vi "Show State State.vi"(8 "error in (no error)":errorcluster, 9 "State Name":string, 10 "Category (Optional)":string, 11 "JKI SM in":refnum<class "JKI SM.lvclass">) -> (0 "error out":errorcluster, 3 "JKI SM out":refnum<class "JKI SM.lvclass">)   [LabVIEW 2013, in "JKI State Machine API.lvlib" / "JKI SM.lvclass"]
uses:
  JKI SM.lvclass
  JKI SM.lvclass/JKI SM.ctl
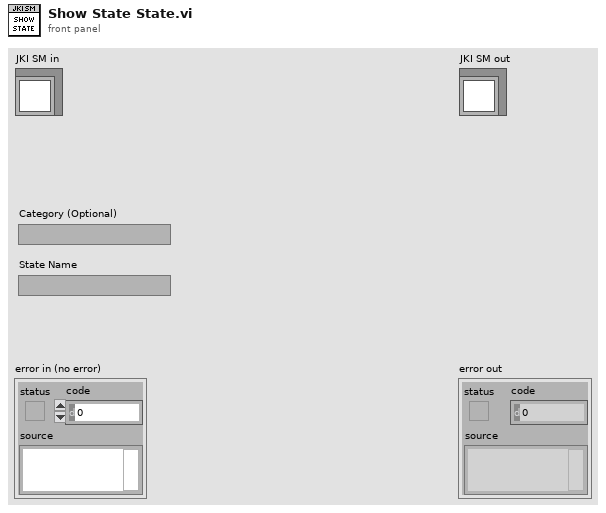
[diagram p1: front panel]
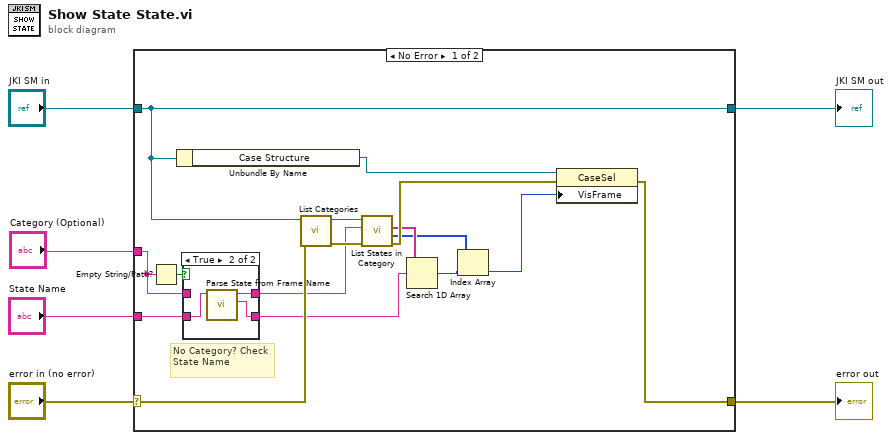
[diagram p0: block diagram]
diagram:
  n1 = case shown="No Error" "error in (no error)" {
    selector: "error in (no error)" -> [w15 w29]
    tunnel: [w22 w29] -> w5
    tunnel: [w16 w28] -> w3
    tunnel: "JKI SM in" -> [w16 w28]
    tunnel: "State Name" -> [w17 _]
    tunnel: "Category (Optional)" -> [w18 _]
    frame No Error {
      # "No Category? Check State Name"
      n2 = Empty String/Path?(string/path=w18) -> (empty?=w19:bool)
      n3 = Unbundle By Name(w16) -> ("Case Structure"=w21:refnum<vi>)
      n4 = case shown="True" w19 {
        tunnel: w17 -> [w23 w27]
        tunnel: [w24 w26] -> w12
        tunnel: w18 -> [w24 _]
        tunnel: [w23 w25] -> w10
        frame False {
        }
        frame True {
          n5 = call "Parse State from Frame Name.vi"("Frame Name"=w27) -> ("State Name"=w25:string, "Category Name"=w26:string)  [unwired: 7 in, 2 out]
        }
      }
      n6 = call "List Categories.vi"("error in (no error)"=w15, "JKI SM in"=w16) -> ("error out"=w14:errorcluster, "JKI SM out"=w13:refnum<class "JKI SM.lvclass">)  [unwired: 6 in, 2 out]
      n7 = call "List States in Category.vi"("error in (no error)"=w14, "Category"=w12, "JKI SM in"=w13) -> ("error out"=w20:errorcluster, "State Frame Indices"=w9:i32[], "States"=w11:string[])  [unwired: 4 in, 2 out]
      n8 = Search 1D Array(1D array=w11, element=w10) -> (index of element=w8:i32)  [unwired: 1 in]
      n9 = Index Array(array=w9, index=w8) -> (element=w7:i32)
      n10 = property class="CaseSel"(reference=w21, error in=w20, "VisFrame"=w7) -> (error out=w22:errorcluster)  [unwired: 1 out]
    }
    frame Error {
    }
  }
  "error out" <- w5
  "JKI SM out" <- w3
